vi "Configure Limit Test.vi"(0 "VISA resource name":refnum<visa-resource-name>, 1 "Lower Limit (0)":dbl, 2 "Auto Clear (F: Disable)":bool, 5 "Function (0: Voltage DC)":i32(ring) items=[" Voltage DC", "Voltage AC", "Current DC", "Current AC", "Resistance", "4-wire Resistance", "Diode", "Capacitance", "Temperature", "Continuity", "Frequency", "Period", "Voltage Ratio", "Digitize Voltage", "Digitize Current"], 7 "Limit Number (1: Limit 1)":i32(ring)=1 items=["Limit 1"=1, "Limit 2"=2], 9 "Channel List(\"\")":string, 11 "error in (no error)":errorcluster, 12 "Upper Limit (0)":dbl, 13 "Enable Limit (F: Disable)":bool) -> (4 "VISA resource name out":refnum<visa-resource-name>, 15 "error out":errorcluster)   [LabVIEW 2023, in "Keithley DMM6500 DAQ6500 Series.lvlib"]
doc: "Configures the limit test."
uses:
  <instrlib>/Keithley DMM6500 DAQ6500 Series/Keithley DMM6500 DAQ6500 Series.lvlib
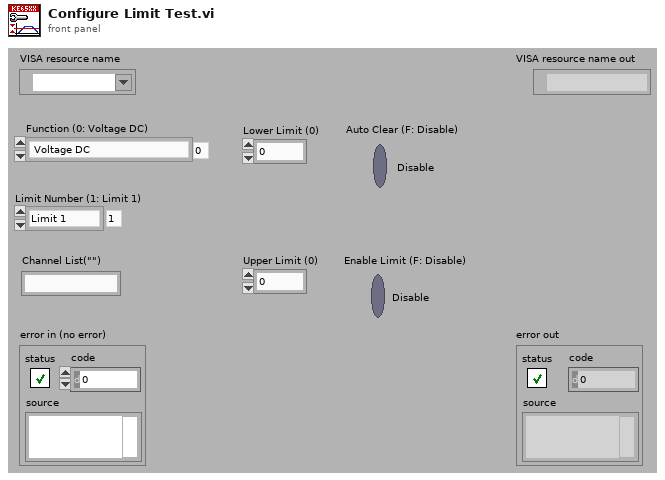
[diagram p1: front panel]
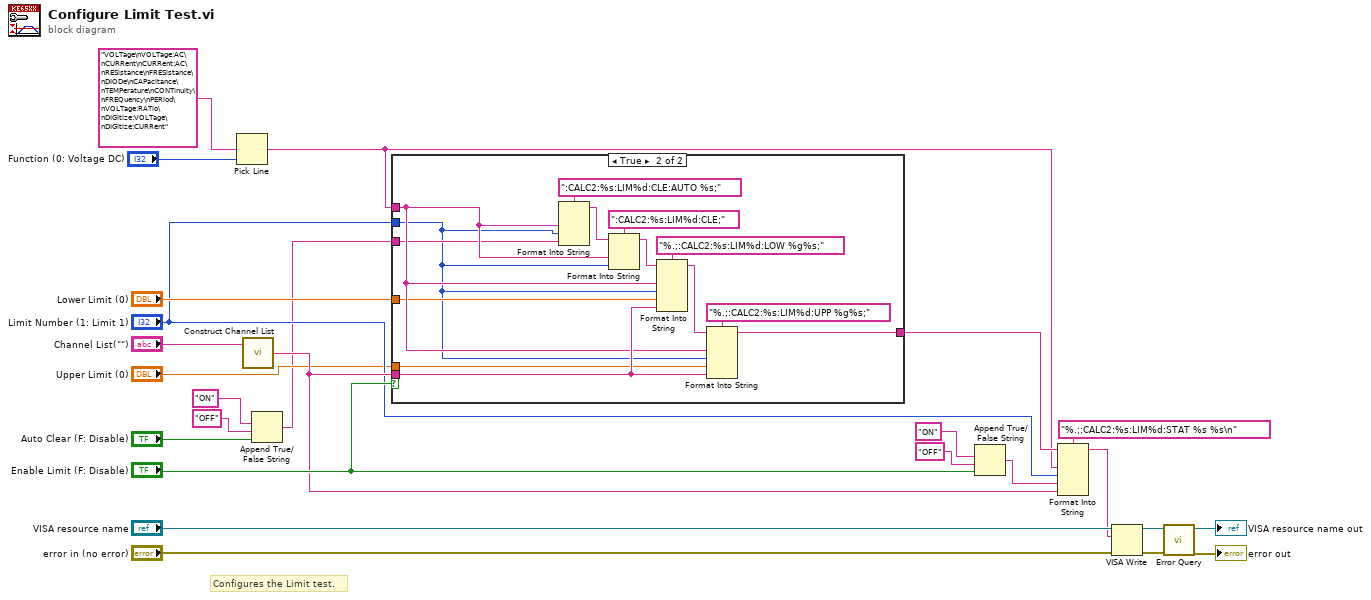
[diagram p0: block diagram]
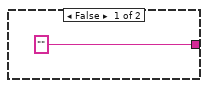
[diagram p2: hidden frame]
diagram:
  # "Configures the Limit test."
  n1 = Pick Line(multi-line string="VOLTage\nVOLTage:AC\nCURRent\nCURRent:AC\nRESistance\nFRESistance\nDIODe\nCAPacitance\nTEMPerature\nCONTinuity\nFREQuency\nPERiod\nVOLTage:RATio\nDIGitize:VOLTage\nDIGitize:CURRent", line index="Function (0: Voltage DC)") -> (output string=w10:string)  [unwired: 1 in]
  n2 = call <instrlib>:"Construct Channel List.vi"("Channel List"="Channel List(\"\")") -> ("Channel List String"=w12:string)  [unwired: 2 in]
  n3 = Append True/False String(1:"Auto Clear (F: Disable)", 2:"OFF", 3:"ON") -> (0:w4:string)  [unwired: 1 in]
  n4 = case shown="True" "Enable Limit (F: Disable)" {
    tunnel: ["" w34] -> w16
    tunnel: w12 -> [_ w32]
    tunnel: "Limit Number (1: Limit 1)" -> [_ w27]
    tunnel: w10 -> [_ w31]
    tunnel: "Lower Limit (0)" -> [_ w30]
    tunnel: "Upper Limit (0)" -> [_ w29]
    tunnel: w4 -> [_ w28]
    frame False {
    }
    frame True {
      n5 = Format Into String(format string=":CALC2:%s:LIM%d:CLE:AUTO %s;", w31, w27, w28) -> (resulting string=w39:string)  [unwired: 2 in, 1 out]
      n6 = Format Into String(format string=":CALC2:%s:LIM%d:CLE;", initial string=w39, w31, w27) -> (resulting string=w33:string)  [unwired: 1 in, 1 out]
      n7 = Format Into String(format string="%.;:CALC2:%s:LIM%d:LOW %g%s;", initial string=w33, w31, w27, w30, w32) -> (resulting string=w36:string)  [unwired: 1 in, 1 out]
      n8 = Format Into String(format string="%.;:CALC2:%s:LIM%d:UPP %g%s;", initial string=w36, w31, w27, w29, w32) -> (resulting string=w34:string)  [unwired: 1 in, 1 out]
    }
  }
  n9 = Append True/False String(1:"Enable Limit (F: Disable)", 2:"OFF", 3:"ON") -> (0:w17:string)  [unwired: 1 in]
  n10 = Format Into String(format string="%.;:CALC2:%s:LIM%d:STAT %s %s\n", initial string=w16, w10, "Limit Number (1: Limit 1)", w17, w12) -> (resulting string=w15:string)  [unwired: 1 in, 1 out]
  n11 = VISA Write(VISA resource name="VISA resource name", write buffer=w15, error in (no error)="error in (no error)") -> (VISA resource name out=w23:refnum<visa-resource-name>, error out=w22:errorcluster)  [unwired: 1 out]
  n12 = call <instrlib>:"Error Query.vi"("error in (no error)"=w22, "VISA resource name"=w23) -> ("error out"=→"error out":errorcluster, "VISA resource name out"=→"VISA resource name out":refnum<visa-resource-name>)  [unwired: 6 in, 2 out]
